vi "C8855-01_OpenCreateReplaceFile.vi"(4 "advisory dialog? (display:T)":bool=TRUE caption="アドバイスダイアログ? (表\\示：T)", 5 "pattern":string="*.xls" caption="パターン", 6 "default name":string caption="デフォルト名", 7 "prompt":string="書き込むファイルを選択。拡張子は自動付加します。" caption="プロンプト", 8 "error in (no error)":errorcluster caption="エラー入力 (エラーなし)", 9 "function (open:0)":T2(ring) caption="関数 (開く：0)", 10 "start path  (Not A Path)":path=path "" caption="開始パス（パスではない）", 11 "file path":path caption="ファイルパス") -> (0 "error out":errorcluster caption="エラー出力", 1 "file size (bytes)":i32 caption="ファイルサイズ（バイト）", 2 "new file path":path caption="新規ファイルパス", 3 "refnum":refnum<file>)   [LabVIEW 2017]
doc: "ファイルダイアログボックスを使用して、プログラム上で、または対話形式で既存ファイルを開いたり、新規ファイルを作成したり、既存ファイルを入れ替えます。"
panel:
  in  "Messages":T1={"Replace existing \"%s\"?"="既存の\"%s\"を置換しますか?", "File \"%s\" exists."="\"%s\"のファイルが存在します。", "Cancel"="キャンセル", "Replace"="置換", "\"%s\" not found."="\"%s\" が見つかりません。", "Open File"="ファイルを開く", "New File"="新規ファイル", "Create File (file exists)"="ファイルを作成（既存ファイル）", "File Dialog"="ファイルダイアログ", "Open or Create File %d"="ファイルを開くまたは作成する(function=%d)", "EOF"="EOF"} caption="メッセージ"
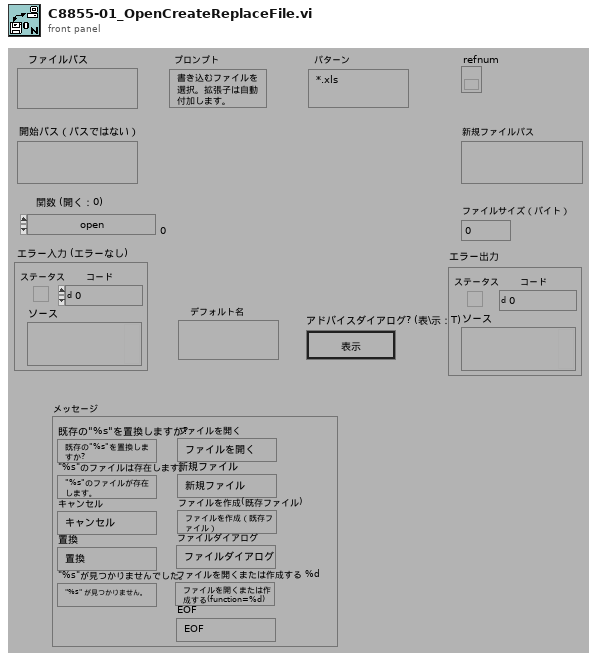
[diagram p1: front panel]
types:
  T1 = cluster{"Replace existing \"%s\"?":string, "File \"%s\" exists.":string, "Cancel":string, "Replace":string, "\"%s\" not found.":string, "Open File":string, "New File":string, "Create File (file exists)":string, "File Dialog":string, "Open or Create File %d":string, "EOF":string}
  T2 = enum16{"open", "open or create", "create or replace", "create", "open (read only)"}
  T3 = enum16{"read/write", "read-only", "write-only", "write-only (truncate)"}
  T4 = enum16{"open", "open or create", "create or replace", "create"}
  T5 = enum16{"open", "replace", "create", "open or create", "replace or create", "replace or create with confirmation"}
  T6 = enum16{"existing file", "new file", "new or existing file", "existing dir", "new dir", "new or existing dir"}[]
  T7 = enum16{"existing file", "new file", "new or existing file", "existing dir", "new dir", "new or existing dir"}
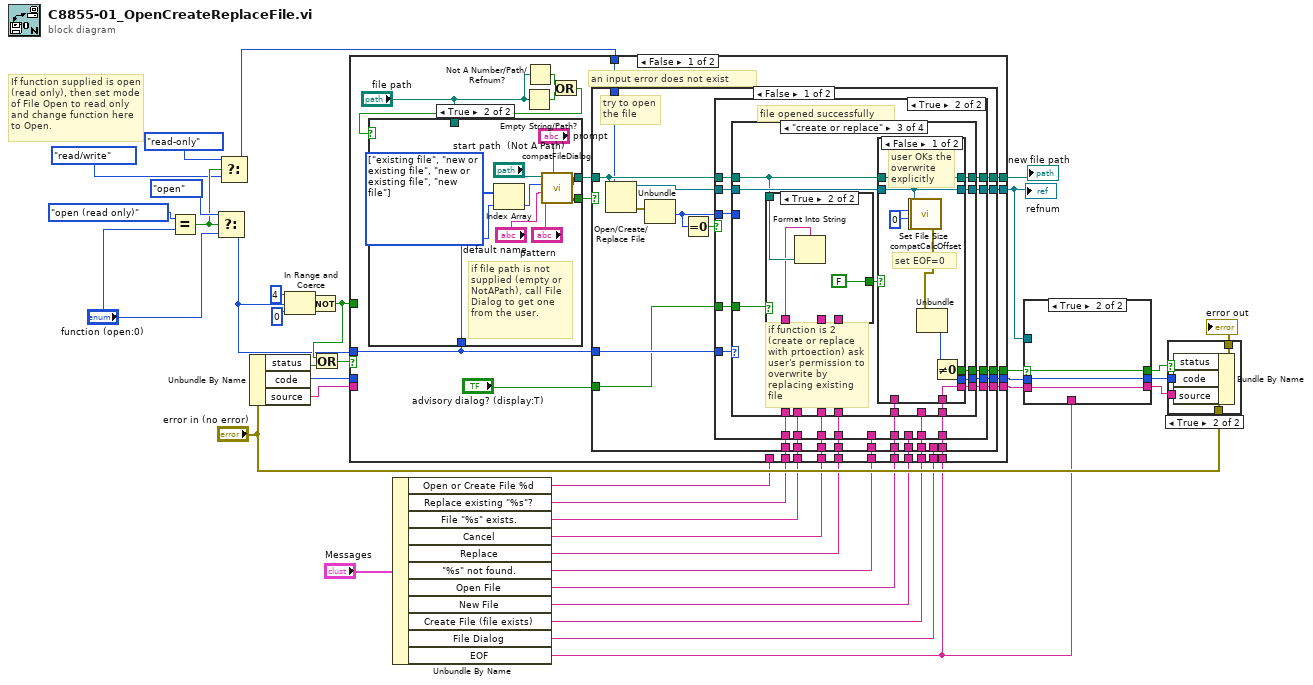
[diagram p0: block diagram]
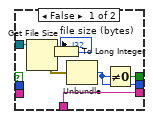
[diagram p3: hidden frame]
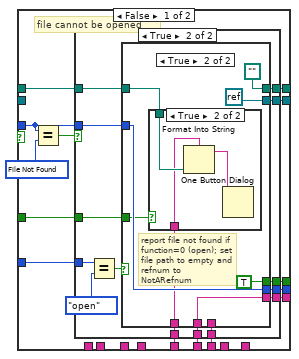
[diagram p4: hidden frame]
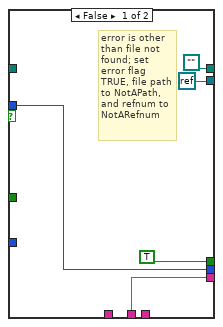
[diagram p5: hidden frame]
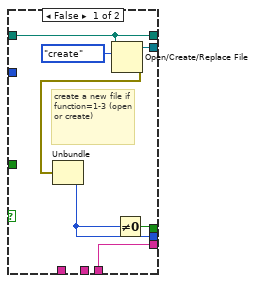
[diagram p6: hidden frame]
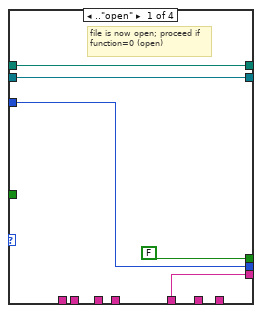
[diagram p8: hidden frame]
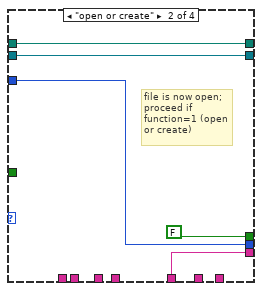
[diagram p9: hidden frame]
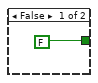
[diagram p10: hidden frame]
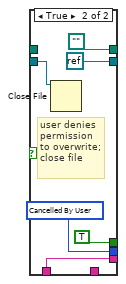
[diagram p11: hidden frame]
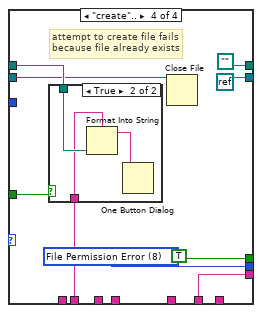
[diagram p12: hidden frame]
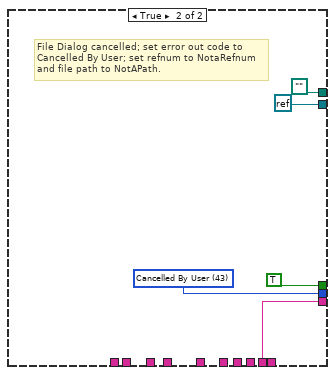
[diagram p14: hidden frame]
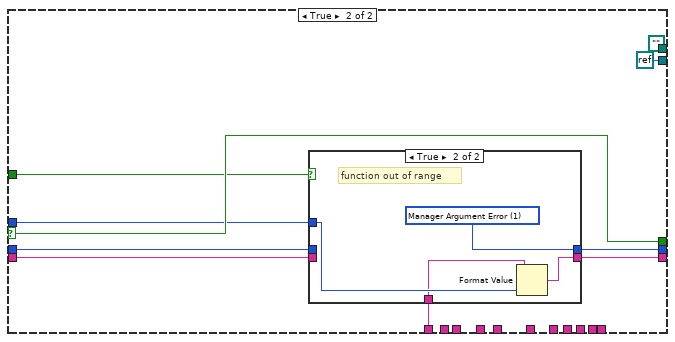
[diagram p16: hidden frame]
diagram:
  # "If function supplied is open (read only), then set mode of File Open to read only and change function here to Open."
  n1 = Equal?(x=T2."open (read only)" ("y"), y="function (open:0)") -> (x = y?=w6:bool)
  n2 = Select(t=T2."open", s=w6, f="function (open:0)") -> (s? t:f=w3:T2)
  n3 = Select(t=T3."read-only" ("open mode (0)"), s=w6, f=T3."read/write" ("open mode (0)")) -> (s? t:f=w1:T3)
  n4 = Unbundle By Name("error in (no error)") -> ("status"=w28:bool, "code"=w27:i32, "source"=w26:string)
  n5 = In Range and Coerce(upper limit=4, x=w3, lower limit=0) -> (In Range?=w33:bool)  [unwired: 1 out]
  n6 = Not(x=w33) -> (.not. x?=w35:bool)
  n7 = Or(x=w35, y=w28) -> (x .or. y?=w34:bool)
  n8 = Unbundle By Name("Messages") -> ("Open or Create File %d"=w10:string, "Replace existing \"%s\"?"=w19:string, "File \"%s\" exists."=w18:string, "Cancel"=w17:string, "Replace"=w16:string, "\"%s\" not found."=w15:string, "Open File"=w14:string, "New File"=w13:string, "Create File (file exists)"=w12:string, "File Dialog"=w11:string, "EOF"=w9:string)
  n9 = case shown="FALSE" w34 {
    selector: w34 -> [_ w232]
    tunnel: [w60 path ""] -> w38
    tunnel: [w59 refnum<k0> refnum] -> w29
    tunnel: [w58 w229] -> w30
    tunnel: [w57 w232] -> w32
    tunnel: [w56 w231] -> w31
    tunnel: w27 -> [_ w230]
    tunnel: w26 -> [_ w228]
    tunnel: w3 -> [w50 w227]
    tunnel: w35 -> [_ w226]
    tunnel: w14 -> [w49 _]
    tunnel: w13 -> [w48 _]
    tunnel: w15 -> [w47 _]
    tunnel: w16 -> [w46 _]
    tunnel: w17 -> [w45 _]
    tunnel: w19 -> [w44 _]
    tunnel: w12 -> [w43 _]
    tunnel: w18 -> [w42 _]
    tunnel: w11 -> [w41 _]
    tunnel: w10 -> [_ w225]
    tunnel: w9 -> [w40 _]
    tunnel: w1 -> [w39 _]
    frame False {
      # "an input error does not exist"
      n10 = Empty String/Path?(string/path="file path") -> (empty?=w53:bool)
      n11 = Not A Number/Path/Refnum?(number/path/refnum="file path") -> (NaN/Path/Refnum?=w54:bool)
      n12 = Or(x=w54, y=w53) -> (x .or. y?=w52:bool)
      n13 = case shown="TRUE" w52 {
        selector: w52 -> [w214 _]
        tunnel: [w214 w222] -> w62
        tunnel: [w215 w221] -> w61
        tunnel: "file path" -> [w215 _]
        tunnel: w50 -> [_ w217]
        frame False {
          # "a File Path is supplied (not empty); proceed"
        }
        frame True {
          w218 = T6 [enum."existing file", enum."new or existing file", enum."new or existing file", enum."new file"] items=["existing file", "new file", "new or existing file", "existing dir", "new dir", "new or existing dir"]
          # "if file path is not supplied (empty or NotAPath), call File Dialog to get one from the user."
          n14 = Index Array(array=w218, index=w217) -> (element=w219:T7)
          n15 = call <vilib>:"compatFileDialog.vi"("prompt"="prompt", "pattern"="pattern", "default name"="default name", "select mode (2)"=w219, "start path"="start path  (Not A Path)") -> ("cancelled"=w222:bool, "path"=w221:path)  [unwired: 2 in, 3 out]
        }
      }
      n16 = case shown="FALSE" w62 {
        tunnel: w61 -> [w83 _]
        tunnel: [w82 path ""] -> w60
        tunnel: w50 -> [w81 _]
        tunnel: [w80 refnum<k0> refnum] -> w59
        tunnel: [w78 w209] -> w58
        tunnel: [w77 TRUE] -> w57
        tunnel: [w76 w212] -> w56
        tunnel: "advisory dialog? (display:T)" -> [w74 _]
        tunnel: w49 -> [w72 _]
        tunnel: w48 -> [w71 _]
        tunnel: w47 -> [w70 _]
        tunnel: w46 -> [w69 _]
        tunnel: w45 -> [w68 _]
        tunnel: w44 -> [w67 _]
        tunnel: w43 -> [w66 _]
        tunnel: w42 -> [w65 _]
        tunnel: w41 -> [_ w209]
        tunnel: w40 -> [w64 _]
        tunnel: w39 -> [w63 _]
        frame False {
          # "try to open the file"
          n17 = Open/Create/Replace File(file path (use dialog)=w83, access (0:read/write)=w63) -> (refnum out=w79:refnum<file>, error out=w84:errorcluster)  [unwired: 1 in, 4 out]
          n18 = Unbundle(w84) -> ("code"=w73:i32)  [unwired: 2 out]
          n19 = Equal To 0?(x=w73) -> (x = 0?=w75:bool)
          n20 = case shown="TRUE" w75 {
            tunnel: w73 -> [w89 w145]
            tunnel: w83 -> [w96 w151]
            tunnel: [w95 w152] -> w82
            tunnel: w81 -> [w94 w144]
            tunnel: [w93 w150] -> w80
            tunnel: w79 -> [_ w149]
            tunnel: [w92 w148] -> w78
            tunnel: [w91 w147] -> w77
            tunnel: [w90 w146] -> w76
            tunnel: w74 -> [w88 w143]
            tunnel: w72 -> [w87 w142]
            tunnel: w71 -> [w86 _]
            tunnel: w70 -> [w85 _]
            tunnel: w69 -> [_ w141]
            tunnel: w68 -> [_ w140]
            tunnel: w67 -> [_ w139]
            tunnel: w66 -> [_ w138]
            tunnel: w65 -> [_ w137]
            tunnel: w64 -> [_ w136]
            frame False {
              w98 = u16 7 items=["No Error", "Manager Argument Error", "Memory Full", "Out of Zone", "End of File", "File Already Open", "Generic File IO Error", "File Not Found", "File Permission Error", "Disk Full", "Duplicate Path", "Too Many Files Open", "Not Enabled", "Resource File Not Found", "Cannot Add Resource", "Resource Not Found", "Image Not Found", "Image Memory Error", "Pen Does Not Exist", "Config Bad Type", "Config Token Not Found", "Config Parse Error", "Config Memory Error", "Bad External Code Format", "Bad External Code Offset", "External Code Not Present", "Null Window", "Destroy Window Mixup", "Null Menu", "Print Aborted", "Bad Print Record", "Print Driver Error", "Windows Error During Print", "Memory Error During Print", "Print Dialog Error", "Generic Print Error", "Invalid Device Refnum", "Device Not Found", "Device Parameter Error", "Device Unit Error", "Can't Open Device", "Device Call Aborted", "Generic Error", "Cancelled By User"]
              # "file cannot be opened"
              n21 = Equal?(x=w89, y=w98) -> (x = y?=w97:bool)
              n22 = case shown="TRUE" w97 {
                tunnel: w96 -> [_ w117]
                tunnel: [path "" w116] -> w95
                tunnel: w94 -> [_ w109]
                tunnel: [refnum<k0> refnum w115] -> w93
                tunnel: [w99 w114] -> w92
                tunnel: [TRUE w113] -> w91
                tunnel: [w100 w112] -> w90
                tunnel: w89 -> [w100 w111]
                tunnel: w88 -> [_ w110]
                tunnel: w87 -> [w99 w105]
                tunnel: w86 -> [_ w106]
                tunnel: w85 -> [_ w104]
                frame False {
                  # "error is other than file not found; set error flag TRUE, file path to NotAPath, and refnum to NotARefnum"
                }
                frame True {
                  n23 = Equal?(x=w109, y=T4."open") -> (x = y?=w108:bool)
                  n24 = case shown="TRUE" w108 {
                    tunnel: w117 -> [w124 w130]
                    tunnel: [w124 path ""] -> w116
                    tunnel: [w123 refnum<k0> refnum] -> w115
                    tunnel: [w119 w126] -> w114
                    tunnel: [w122 TRUE] -> w113
                    tunnel: [w120 w131] -> w112
                    tunnel: w111 -> [_ w131]
                    tunnel: w110 -> [_ w127]
                    tunnel: w106 -> [w119 _]
                    tunnel: w105 -> [_ w126]
                    tunnel: w104 -> [_ w125]
                    frame False {
                      # "create a new file if function=1-3 (open or create)"
                      n25 = Open/Create/Replace File(file path (use dialog)=w124, operation (0:open)=T5."create" ("操作 (0:開く)")) -> (refnum out=w123:refnum<file>, error out=w121:errorcluster)  [unwired: 1 in, 4 out]
                      n26 = Unbundle(w121) -> ("code"=w120:i32)  [unwired: 2 out]
                      n27 = Not Equal To 0?(x=w120) -> (x != 0?=w122:bool)
                    }
                    frame True {
                      # "report file not found if function=0 (open); set file path to empty and refnum to NotARefnum"
                      n28 = case shown="TRUE" w127 {
                        tunnel: w130 -> [_ w135]
                        tunnel: w125 -> [_ w134]
                        frame False {
                        }
                        frame True {
                          n29 = Format Into String(format string=w134, w135) -> (resulting string=w133:string)  [unwired: 2 in, 1 out]
                          n30 = One Button Dialog(message=w133) -> ()  [unwired: 2 out]
                        }
                      }
                    }
                  }
                }
              }
            }
            frame True {
              # "file opened successfully"
              n31 = case shown="\"create or replace\"" w144 {
                tunnel: [w157 w159 w176 path ""] -> w152
                tunnel: w151 -> [w157 w159 w168 w205]
                tunnel: [w156 w160 w175 refnum<k0> refnum] -> w150
                tunnel: w149 -> [w156 w160 w174 w202]
                tunnel: [w153 w158 w173 w198] -> w148
                tunnel: [FALSE FALSE w172 TRUE] -> w147
                tunnel: [w154 w162 w171 w203] -> w146
                tunnel: w145 -> [w154 w162 _ _]
                tunnel: w143 -> [_ _ w169 w204]
                tunnel: w142 -> [w153 w158 w164 _]
                tunnel: w141 -> [_ _ w167 _]
                tunnel: w140 -> [_ _ w166 _]
                tunnel: w139 -> [_ _ w165 _]
                tunnel: w138 -> [_ _ _ w198]
                tunnel: w137 -> [_ _ _ w197]
                tunnel: w136 -> [_ _ w163 _]
                frame .."open" {
                  # "file is now open; proceed if function=0 (open)"
                }
                frame "open or create" {
                  # "file is now open; proceed if function=1 (open or create)"
                }
                frame "create or replace" {
                  # "if function is 2 (create or replace with prtoection) ask user's permission to overwrite by replacing existing file"
                  n32 = case shown="TRUE" w169 {
                    tunnel: [FALSE FALSE] -> w170
                    tunnel: w168 -> [_ w179]
                    tunnel: w167 -> [_ _]
                    tunnel: w166 -> [_ _]
                    tunnel: w165 -> [_ w178]
                    frame False {
                    }
                    frame True {
                      n33 = Format Into String(format string=w178, w179) -> ()  [unwired: 2 in, 2 out]
                    }
                  }
                  n34 = case shown="FALSE" w170 {
                    tunnel: [w186 path ""] -> w176
                    tunnel: [w190 refnum<k0> refnum] -> w175
                    tunnel: w174 -> [w190 w194]
                    tunnel: [w184 w191] -> w173
                    tunnel: [w188 TRUE] -> w172
                    tunnel: [w185 w192] -> w171
                    tunnel: w168 -> [w186 _]
                    tunnel: w164 -> [_ w191]
                    tunnel: w163 -> [w184 _]
                    frame False {
                      w189 = 0
                      # "set EOF=0"
                      # "user OKs the overwrite explicitly"
                      n35 = call <vilib>:"compatCalcOffset.vi"("pos offset (0)"=w189, "pos mode (0:1)"=w189, "refnum"=w190) -> ("error out"=w183:errorcluster, "offset"=w182:i32, "dup refnum"=w181:refnum<file>)  [unwired: 1 in, 5 out]
                      n36 = Set File Size(4:w183, 6:w182, 7:w181) -> (0:w187:errorcluster)  [unwired: 1 out]
                      n37 = Unbundle(w187) -> ("code"=w185:i32)  [unwired: 2 out]
                      n38 = Not Equal To 0?(x=w185) -> (x != 0?=w188:bool)
                    }
                    frame True {
                      w192 = u16 43 items=["No Error", "Manager Argument Error", "Memory Full", "Out of Zone", "End of File", "File Already Open", "Generic File IO Error", "File Not Found", "File Permission Error", "Disk Full", "Duplicate Path", "Too Many Files Open", "Not Enabled", "Resource File Not Found", "Cannot Add Resource", "Resource Not Found", "Image Not Found", "Image Memory Error", "Pen Does Not Exist", "Config Bad Type", "Config Token Not Found", "Config Parse Error", "Config Memory Error", "Bad External Code Format", "Bad External Code Offset", "External Code Not Present", "Null Window", "Destroy Window Mixup", "Null Menu", "Print Aborted", "Bad Print Record", "Print Driver Error", "Windows Error During Print", "Memory Error During Print", "Print Dialog Error", "Generic Print Error", "Invalid Device Refnum", "Device Not Found", "Device Parameter Error", "Device Unit Error", "Can't Open Device", "Device Call Aborted", "Generic Error", "Cancelled By User"]
                      # "user denies permission to overwrite; close file"
                      n39 = Close File(refnum=w194) -> ()  [unwired: 1 in, 2 out]
                    }
                  }
                }
                frame "create".. {
                  w203 = u16 8 items=["No Error", "Argument Error", "Memory Full", "Out of Zone", "End of File", "File Already Open", "Generic File IO Error", "File Not Found", "File Permission Error", "Disk Full", "Duplicate Path", "Too Many Files Open", "Not Enabled", "Resource File Not Found", "Cannot Add Resource", "Resource Not Found", "Image Not Found", "Image Memory Error", "Pen Does Not Exist", "Config Bad Type", "Config Token Not Found", "Config Parse Error", "Config Memory Error", "Bad External Code Format", "Bad External Code Offset", "External Code Not Present", "Null Window", "Destroy Window Mixup", "Null Menu", "Print Aborted", "Bad Print Record", "Print Driver Error", "Windows Error During Print", "Memory Error During Print", "Print Dialog Error", "Generic Print Error", "Invalid Device Refnum", "Device Not Found", "Device Parameter Error", "Device Unit Error", "Can't Open Device", "Device Call Aborted", "Generic Error", "Cancelled By User", "Object ID Too Low", "Object ID Too High", "Object Not In Heap", "Unknown Heap", "Bad DefProc ID", "DefProc Not In Table", "Message Out Of Range", "Null Method", "Unknown Message", "Manager Call Not Supported", "Bad address", "Connection In progress", "Connection timed out", "Connection is already in progress", "Network attribute not supported", "Network error", "Address in use", "System out of memory", "Connection aborted", "Connection refused", "Connection is not connected", "Connection is already connected", "Connection closed", "Initialize error (interapplication manager)", "Bad occurrence", "Wait on unbound occurrence handler", "Occurrence queue overflow", "Bad path", "Semaphore not signaled", "Unrecognized type (interapplication manager)"]
                  # "attempt to create file fails because file already exists"
                  n40 = case shown="TRUE" w204 {
                    tunnel: w205 -> [_ w208]
                    tunnel: w197 -> [_ w206]
                    frame False {
                    }
                    frame True {
                      n41 = Format Into String(format string=w206, w208) -> (resulting string=w207:string)  [unwired: 2 in, 1 out]
                      n42 = One Button Dialog(message=w207) -> ()  [unwired: 2 out]
                    }
                  }
                  n43 = Close File(refnum=w202) -> ()  [unwired: 1 in, 2 out]
                }
              }
            }
          }
        }
        frame True {
          w212 = u16 43 items=["No Error", "Manager Argument Error", "Memory Full", "Out of Zone", "End of File", "File Already Open", "Generic File IO Error", "File Not Found", "File Permission Error", "Disk Full", "Duplicate Path", "Too Many Files Open", "Not Enabled", "Resource File Not Found", "Cannot Add Resource", "Resource Not Found", "Image Not Found", "Image Memory Error", "Pen Does Not Exist", "Config Bad Type", "Config Token Not Found", "Config Parse Error", "Config Memory Error", "Bad External Code Format", "Bad External Code Offset", "External Code Not Present", "Null Window", "Destroy Window Mixup", "Null Menu", "Print Aborted", "Bad Print Record", "Print Driver Error", "Windows Error During Print", "Memory Error During Print", "Print Dialog Error", "Generic Print Error", "Invalid Device Refnum", "Device Not Found", "Device Parameter Error", "Device Unit Error", "Can't Open Device", "Device Call Aborted", "Generic Error", "Cancelled By User"]
          # "File Dialog cancelled; set error out code to Cancelled By User; set refnum to NotaRefnum and file path to NotAPath."
        }
      }
    }
    frame True {
      n44 = case shown="TRUE" w226 {
        tunnel: [w236 w240] -> w231
        tunnel: w230 -> [w236 _]
        tunnel: [w235 w239] -> w229
        tunnel: w228 -> [w235 _]
        tunnel: w227 -> [_ w238]
        tunnel: w225 -> [_ w237]
        frame False {
          # "on an input error, do nothing"
        }
        frame True {
          w240 = u16 1 items=["No Error", "Manager Argument Error", "Memory Full", "Out of Zone", "End of File", "File Already Open", "Generic File IO Error", "File Not Found", "File Permission Error", "Disk Full", "Duplicate Path", "Too Many Files Open", "Not Enabled", "Resource File Not Found", "Cannot Add Resource", "Resource Not Found", "Image Not Found", "Image Memory Error", "Pen Does Not Exist", "Config Bad Type", "Config Token Not Found", "Config Parse Error", "Config Memory Error", "Bad External Code Format", "Bad External Code Offset", "External Code Not Present", "Null Window", "Destroy Window Mixup", "Null Menu", "Print Aborted", "Bad Print Record", "Print Driver Error", "Windows Error During Print", "Memory Error During Print", "Print Dialog Error", "Generic Print Error", "Invalid Device Refnum", "Device Not Found", "Device Parameter Error", "Device Unit Error", "Can't Open Device", "Device Call Aborted", "Generic Error", "Cancelled By User"]
          # "function out of range"
          n45 = Format Value(format string=w237, value (0)=w238) -> (output string=w239:string)  [unwired: 1 out]
        }
      }
    }
  }
  "new file path" <- w38
  "refnum" <- w29
  n46 = case shown="TRUE" w32 {
    selector: w32 -> [_ w250]
    tunnel: w31 -> [_ w249]
    tunnel: w30 -> [_ w248]
    tunnel: [w247 w250] -> w25
    tunnel: [w244 w249] -> w24
    tunnel: [w242 w248] -> w23
    tunnel: w29 -> [w246 _]
    tunnel: w9 -> [w242 _]
    frame False {
      n47 = Get File Size(file=w246) -> (size (in bytes)=w241:i64, 0:w243:errorcluster)  [unwired: 1 in, 1 out]
      n48 = To Long Integer(number=w241) -> (32bit integer=→"file size (bytes)":i32)
      n49 = Unbundle(w243) -> ("code"=w244:i32)  [unwired: 2 out]
      n50 = Not Equal To 0?(x=w244) -> (x != 0?=w247:bool)
    }
    frame True {
    }
  }
  n51 = case shown="TRUE" w25 {
    selector: w25 -> [_ w255]
    tunnel: w24 -> [_ w256]
    tunnel: w23 -> [_ w254]
    tunnel: "error in (no error)" -> [w251 w253]
    tunnel: [w251 w252] -> w21
    frame False {
    }
    frame True {
      n52 = Bundle By Name(cluster=w253, "status"=w255, "code"=w256, "source"=w254) -> (w252:errorcluster)
    }
  }
  "error out" <- w21
